vi "Initialize.vi"(8 "error in (no error)":errorcluster, 9 "Reset (True)":bool=TRUE, 10 "ID Query (True)":bool=TRUE, 11 "VISA resource name":refnum<visa-resource-name>) -> (0 "error out":errorcluster, 3 "VISA resource name out":refnum<visa-resource-name>)   [LabVIEW 2009, in "Agilent 81150.lvlib"]
doc: "Establishes communication with the instrument and optionally performs an instrument identification query and/or an instrument reset. It also places the instrument in a default state needed for other instrument driver operations. Therefore, call this VI before calling other instrument driver VIs for this instrument. Generally, you need to call the Initialize VI only once at the beginning of an application."
uses:
  Agilent 81150.lvlib
panel:
  # "(c) 2008-2013 National Instruments.  ALL RIGHTS RESERVED."
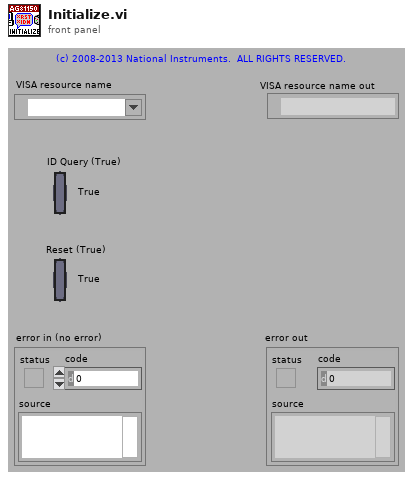
[diagram p1: front panel]
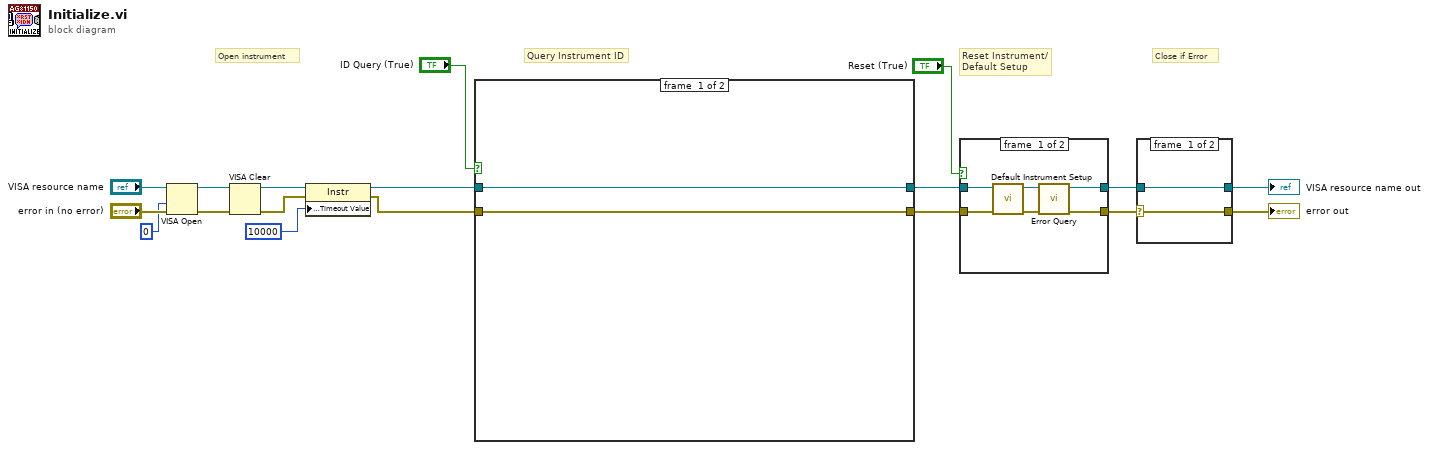
[diagram p0: block diagram]
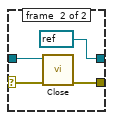
[diagram p2: hidden frame]
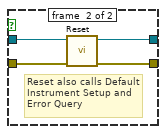
[diagram p3: hidden frame]
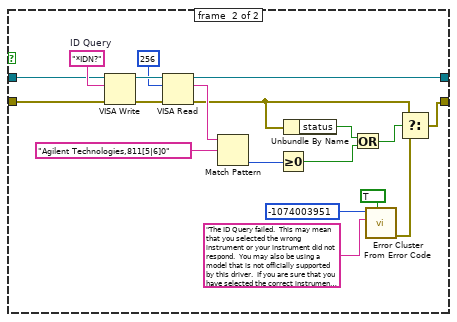
[diagram p4: hidden frame]
diagram:
  # "Close if Error"
  # "Query Instrument ID"
  # "Reset Instrument/\nDefault Setup"
  # "Open instrument"
  n1 = VISA Open(access mode=u32 0, error in (no error)="error in (no error)", VISA resource name="VISA resource name") -> (VISA resource name=w10:refnum<visa-resource-name>, error out=w9:errorcluster)  [unwired: 2 out]
  n2 = VISA Clear(VISA resource name=w10, error in (no error)=w9) -> (VISA resource name out=w8:refnum<visa-resource-name>, error out=w7:errorcluster)
  n3 = property class="Instr"(reference=w8, error in=w7, "General Settings:Timeout Value"=u32 10000) -> (reference out=w2:refnum<visa-resource-name>, error out=w1:errorcluster)
  n4 = case shown="True" "ID Query (True)" {
    tunnel: [w19 w39] -> w17
    tunnel: [w20 w38] -> w18
    tunnel: w2 -> [w20 w22]
    tunnel: w1 -> [w19 w21]
    frame #0 {
    }
    frame #1 {
      w32 = "*IDN?"  # ID Query
      n5 = VISA Write(VISA resource name=w22, write buffer=w32, error in (no error)=w21) -> (VISA resource name out=w36:refnum<visa-resource-name>, error out=w35:errorcluster)  [unwired: 1 out]
      n6 = VISA Read(VISA resource name=w36, byte count=u32 256, error in (no error)=w35) -> (VISA resource name out=w38:refnum<visa-resource-name>, read buffer=w37:string, error out=w26:errorcluster)  [unwired: 1 out]
      n7 = Match Pattern(string=w37, regular expression="Agilent Technologies,811[5|6]0") -> (offset past match=w27:i32)  [unwired: 4 out]
      n8 = Greater Or Equal To 0?(x=w27) -> (x >= 0?=w24:bool)
      n9 = Unbundle By Name(w26) -> ("status"=w25:bool)
      n10 = Or(x=w25, y=w24) -> (x .or. y?=w23:bool)
      n11 = call <vilib>:"Error Cluster From Error Code.vi"("show call chain? (False)"=TRUE, "error message (\"\")"="The ID Query failed.  This may mean that you selected the wrong instrument or your instrument did not respond.  You may also be using a model that is not officially supported by this driver.  If you are sure that you have selected the correct instrument and it is responding, try disabling the ID Query." ("Source (VI Name)"), "error code (0)"=-1074003951 ("Code")) -> ("error out"=w31:errorcluster)  [unwired: 1 in, 5 out]
      n12 = Select(t=w26, s=w23, f=w31) -> (s? t:f=w39:errorcluster)
    }
  }
  n13 = case shown="True" "Reset (True)" {
    tunnel: w17 -> [w44 w46]
    tunnel: [w41 w49] -> w3
    tunnel: w18 -> [w45 w47]
    tunnel: [w42 w48] -> w4
    frame #0 {
      n14 = call "Default Instrument Setup.vi"("error in (no error)"=w44, "VISA resource name"=w45) -> ("error out"=w40:errorcluster, "VISA resource name out"=w43:refnum<visa-resource-name>)  [unwired: 8 out]
      n15 = call "Error Query.vi"("error in (no error)"=w40, "VISA resource name"=w43) -> ("error out"=w41:errorcluster, "VISA resource name out"=w42:refnum<visa-resource-name>)  [unwired: 8 out]
    }
    frame #1 {
      # "Reset also calls Default Instrument Setup and Error Query"
      n16 = call "Reset.vi"("error in (no error)"=w46, "VISA resource name"=w47) -> ("error out"=w49:errorcluster, "VISA resource name out"=w48:refnum<visa-resource-name>)  [unwired: 8 out]
    }
  }
  n17 = case shown="Error" w3 {
    selector: w3 -> [w50 w53]
    tunnel: w4 -> [w51 w54]
    tunnel: [w51 refnum<visa-resource-name> refnum ("VISA resource name out")] -> w6
    tunnel: [w50 w55] -> w5
    frame #0 {
    }
    frame #1 {
      n18 = call "Close.vi"("error in (no error)"=w53, "VISA resource name"=w54) -> ("error out"=w55:errorcluster)  [unwired: 9 out]
    }
  }
  "VISA resource name out" <- w6
  "error out" <- w5
